vi "4461 - Get Cal Info.vi"(8 "error in (no error)":errorcluster, 11 "Lockin":refnum<class "Instrument.Lockin.lvclass">) -> (0 "error out":errorcluster, 2 "Cal Info":T1(array[cluster]), 3 "Lockkin out":refnum<class "Instrument.Lockin.lvclass">)   [LabVIEW 2016, in "Instrument.Lockin.lvclass"]
uses:
  Instrument.Lockin.lvclass
  Instrument.Lockin.lvclass/Instrument.Lockin.ctl
  <userlib>/_OpenG.lib/array/array.llb/Remove Duplicates from 1D Array (String)__ogtk.vi
  <resource>/objmgr/daqmx.rc
panel:
  out "dev temp >5°C from cal temp":bool
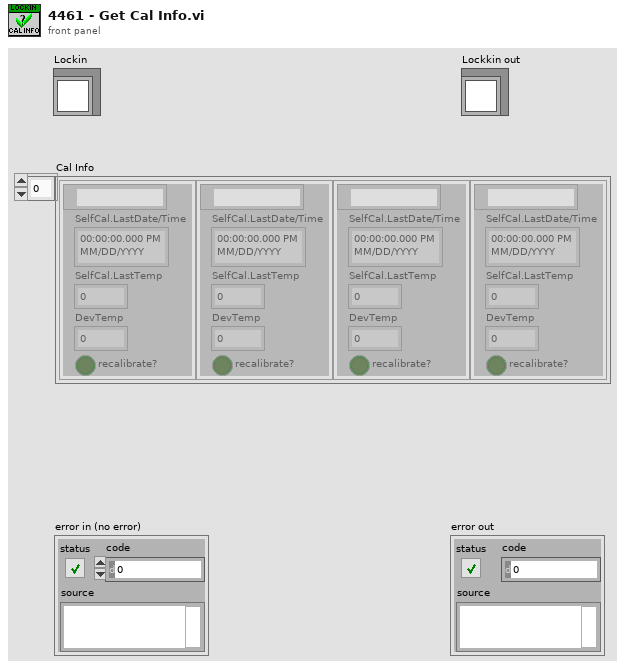
[diagram p1: front panel]
types:
  T1 = cluster{tag, "SelfCal.LastDate/Time":timestamp, "SelfCal.LastTemp":dbl, "DevTemp":dbl, "recalibrate?":bool}[]
  T2 = cluster{"String":string, "SelfCal.LastDate/Time":timestamp, "SelfCal.LastTemp":dbl, "DevTemp":dbl, bool}
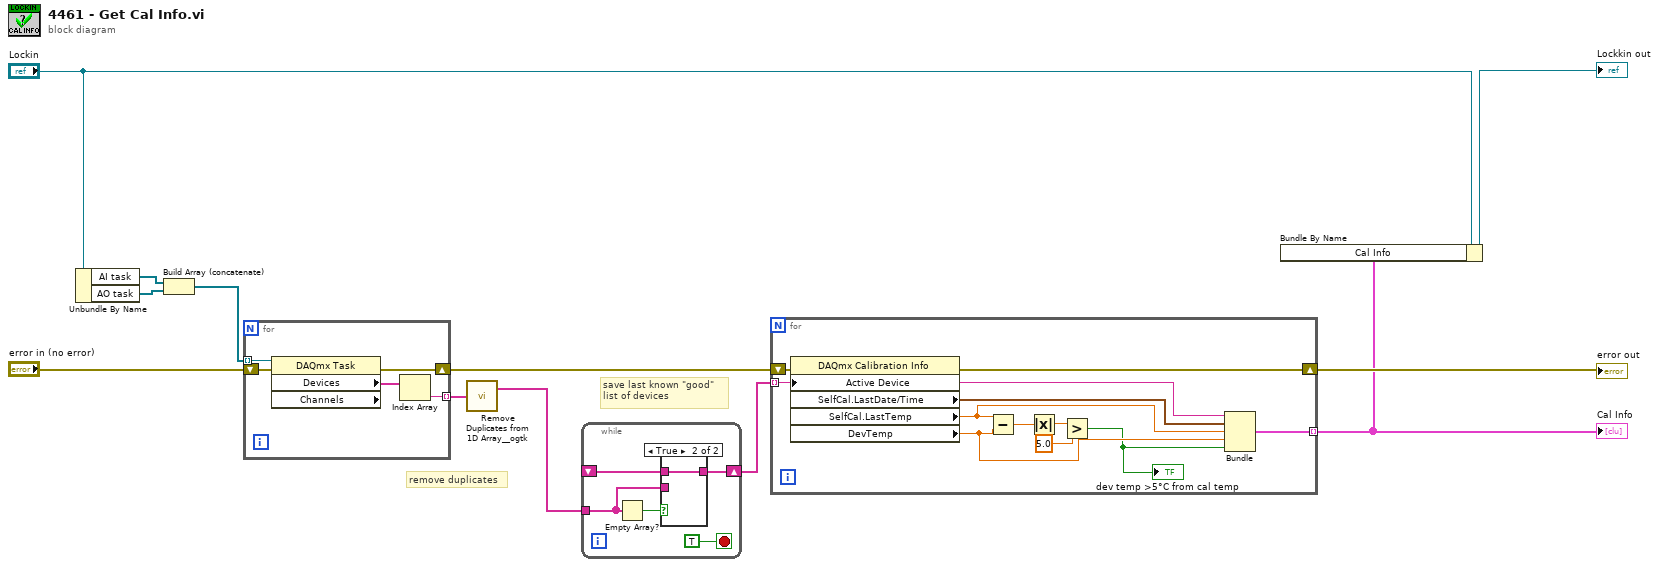
[diagram p0: block diagram]
diagram:
  # "save last known \"good\"\nlist of devices"
  # "remove duplicates"
  n1 = Unbundle By Name("Lockin") -> ("AI task"=w6:refnum<k21>[], "AO task"=w5:refnum<k21>[])
  n2 = Build Array (concatenate)(w6, w5) -> (w11:refnum<k21>[])
  n3 = for {
    tunnel: [w15] -> w10 mode=indexing
    shift-right: [w16] -> w8
    shift-left: "error in (no error)" -> [w17]
    tunnel: w11 -> [w13] mode=indexing
    n4 = property class="DAQmx Task" props=["Devices", "Channels"](reference=w13, error in=w17) -> (error out=w16:errorcluster, "Devices"=w14:tag[])  [unwired: 2 out]
    n5 = Index Array(array=w14) -> (element=w15:tag)  [unwired: 1 in]
  }
  n6 = call-poly <userlib>:"Remove Duplicates from 1D Array__ogtk.vi"("Input Array"=w10) -> ("Output Array"=w2:string[])  [unwired: 1 out]
  n7 = while {
    shift-right: [w20] -> w7
    shift-left: _ -> [w18]
    tunnel: w2 -> [w19]
    stop <- TRUE stop-if-true
    n8 = Empty Array?(array=w19) -> (empty?=w21:bool)
    n9 = case shown="True" w21 {
      tunnel: [w23 w24] -> w20
      tunnel: w19 -> [w23 _]
      tunnel: w18 -> [_ w24]
      frame False {
      }
      frame True {
      }
    }
  }
  n10 = for {
    tunnel: [w34] -> w1 mode=indexing
    shift-right: [w35] -> w9
    shift-left: w8 -> [w33]
    tunnel: w7 -> [w25] mode=indexing
    n11 = property class="DAQmx Calibration Info"(error in=w33, "Active Device"=w25) -> (error out=w35:errorcluster, "SelfCal.LastDate/Time"=w29:timestamp, "SelfCal.LastTemp"=w28:dbl, "DevTemp"=w27:dbl)  [unwired: 1 in, 1 out]
    n12 = Subtract(x=w28, y=w27) -> (x-y=w32:dbl)
    n13 = Absolute Value(x=w32) -> (abs(x)=w31:dbl)
    n14 = Greater?(x=w31, y=5.0) -> (0:w26:bool)
    "dev temp >5°C from cal temp" <- w26
    n15 = Bundle("String"=w25, "SelfCal.LastDate/Time"=w29, "SelfCal.LastTemp"=w28, "DevTemp"=w27, w26) -> (w34:T2)  [unwired: 1 in]
  }
  "error out" <- w9
  "Cal Info" <- w1
  n16 = Bundle By Name(cluster="Lockin", "Cal Info"=w1) -> (→"Lockkin out":refnum<class "Instrument.Lockin.lvclass">)
